vi "240112_LabView_with_Lib.vi"   [LabVIEW 2022 SP3]
uses:
  E:/School/AIIT/5AHME/LabView/240112_LabView_with_Lib/231020_Lib_Linear_Interpolation.dll
  231020_Lib_Linear_Interpolation.dll
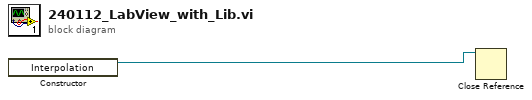
[diagram p0: block diagram]
diagram:
  n1 = constructor class="Interpolation"() -> (reference out=w1:refnum<k24>)  [unwired: 3 in, 2 out]
  n2 = Close Reference(reference=w1) -> ()  [unwired: 1 in, 1 out]
